vi "Initialize.vi"(8 "error in (no error)":errorcluster, 11 "NHRDCPower in":refnum<class "NHRDCPower.lvclass">) -> (0 "error out":errorcluster, 3 "NHRDCPower out":refnum<class "NHRDCPower.lvclass">)   [LabVIEW 2018, in "AcPwrPlugins.lvlib" / "NHRDCPower.lvclass"]
doc: "This VI establishes communication to the instrument and may provide other functions such as reseting the instrument or providing a range check."
uses:
  NHRDCPower.lvclass
  <instrlib>/NHRDCPowerModule/NHRDCPowerModule/NHRDCPowerModule.lvlib
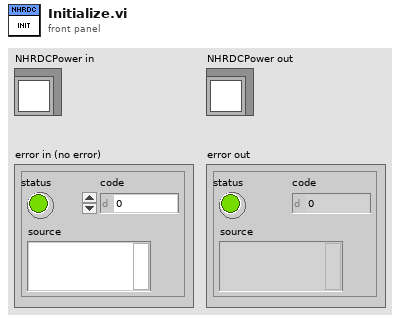
[diagram p1: front panel]
types:
  T1 = cluster{"f":bool, "instrument handle out":refnum<visa-resource-name>}[]
  T2 = typedef "AcPwrPlugins.lvlib/NHRDCPower.lvclass/Device(s)Settings.ctl" = cluster{"MeasName":string, "Modules":T3}
  T3 = typedef "AcPwrPlugins.lvlib/NHRDCPower.lvclass/Modules.ctl" = cluster{"Handle":string, "Name":string, "id query (Yes)":bool, "reset device (Yes)":bool, "Connected":bool, "Initial Battery Detect Voltage (0)":dbl, "SafetySettings":cluster{"SetWatchDog?":bool, "Voltage (V)":dbl, "Current (A)":dbl, "Power (W)":dbl, "Voltage Delay (s)":dbl, "Current Delay (s)":dbl, "Power Delay (s)":dbl}, "Options String":string, "Aperture Time (s)":dbl, "operating state (Off)":i32, "OutputSettings":cluster{"Voltage (V)":dbl, "Current (A)":dbl, "Resistance (Ohms)":dbl, "Power (W)":dbl, "Enable Voltage":bool, "Enable Current":bool, "Enable Resistance":bool, "Enable Power":bool, "Macro After Step Delay  (s)":dbl, "Wait Value (V, A, W)":dbl, "Enable Wait":bool, "Wait on Value":i32}[], "SlewRate":cluster{"Set Voltage Rate V/S":dbl, "Set Current Rate A/S":dbl, "Set Resistance Rate R/S":dbl, "Set Power Rate W/S":dbl}, "Macro":cluster{"Save Macro?":bool, "Load Macro From File?":bool, "Run Macro Continuously?":bool, "Use Macros?":bool, "Load Macro File Path":string, "Save Macro File Path":string}, "Regulation Gain (1=100%)":dbl, "UpdatingOntheFly":bool}[]
  T4 = typedef "AcPwrPlugins.lvlib/NHRDCPower.lvclass/Measurements.ctl" = cluster{"Handle":string, "Name":string, "Enabled":bool, "Measurement Value":sgl, "Measurement Type":enum16{"Power", "Current", "Voltage"}}[]
  T5 = cluster{"Handle Connected?":bool, "Instrument Handle":refnum<visa-resource-name>}
  T6 = cluster{"Handle Connected?":bool, "Instrument Handle":refnum<visa-resource-name>}[]
  T7 = cluster{"Handle":string, "Name":string, "id query (Yes)":bool, "reset device (Yes)":bool, "Connected":bool, "Initial Battery Detect Voltage (0)":dbl, "SafetySettings":cluster{"SetWatchDog?":bool, "Voltage (V)":dbl, "Current (A)":dbl, "Power (W)":dbl, "Voltage Delay (s)":dbl, "Current Delay (s)":dbl, "Power Delay (s)":dbl}, "Options String":string, "Aperture Time (s)":dbl, "operating state (Off)":i32, "OutputSettings":cluster{"Voltage (V)":dbl, "Current (A)":dbl, "Resistance (Ohms)":dbl, "Power (W)":dbl, "Enable Voltage":bool, "Enable Current":bool, "Enable Resistance":bool, "Enable Power":bool, "Macro After Step Delay  (s)":dbl, "Wait Value (V, A, W)":dbl, "Enable Wait":bool, "Wait on Value":i32}[], "SlewRate":cluster{"Set Voltage Rate V/S":dbl, "Set Current Rate A/S":dbl, "Set Resistance Rate R/S":dbl, "Set Power Rate W/S":dbl}, "Macro":cluster{"Save Macro?":bool, "Load Macro From File?":bool, "Run Macro Continuously?":bool, "Use Macros?":bool, "Load Macro File Path":string, "Save Macro File Path":string}, "Regulation Gain (1=100%)":dbl, "UpdatingOntheFly":bool}
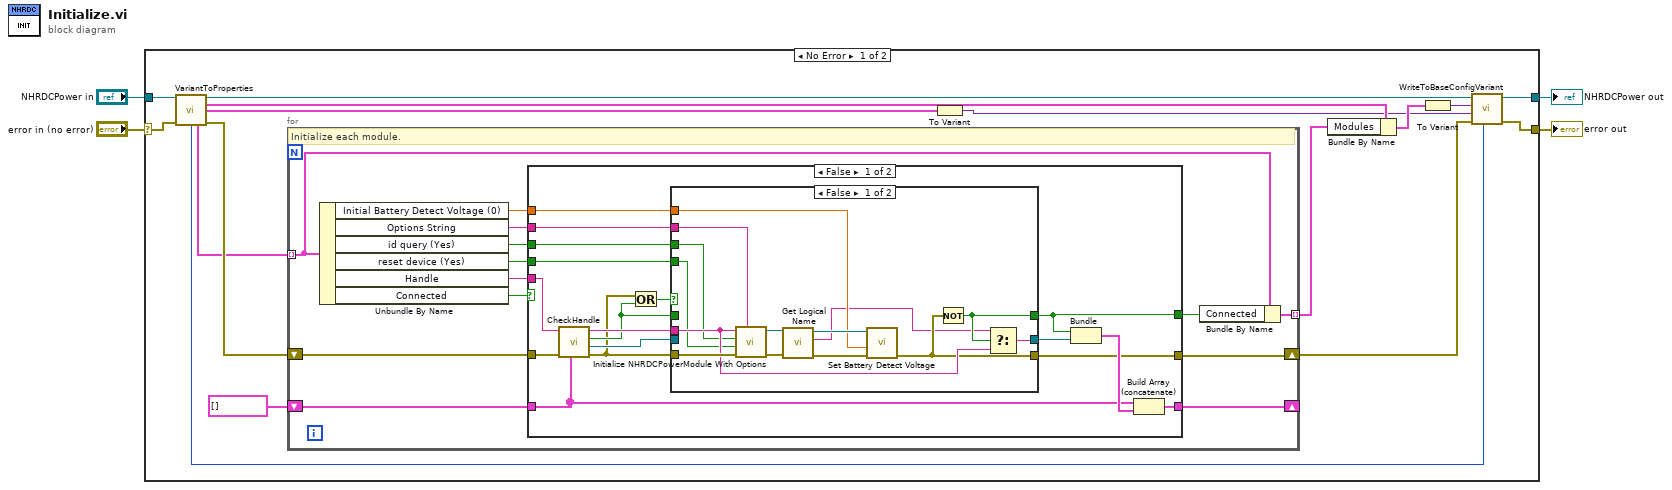
[diagram p0: block diagram]
diagram:
  n1 = case shown="No Error" "error in (no error)" {
    selector: "error in (no error)" -> [w18 w71]
    tunnel: "NHRDCPower in" -> [w17 w72]
    tunnel: [w14 w72] -> w2
    tunnel: [w13 w71] -> w1
    frame No Error {
      n2 = call "VariantToProperties.vi"("NHRDCPower in"=w17, "error in (no error)"=w18) -> ("NHRDCPower out"=w15:refnum<class "NHRDCPower.lvclass">, "NHRDC"=w11:T2, "Meas"=w5:T4, "Measurement Refresh Time (ms)"=w8:u32, "Modules"=w12:T3, "error out"=w19:errorcluster)  [unwired: 7 in, 1 out]
      n3 = for {
        shift-right: [w32] -> w16
        shift-left: w19 -> [w33]
        tunnel: w12 -> [w26] mode=indexing
        shift-right: [w30] -> _
        shift-left: T1 [] -> [w31]
        tunnel: [w25] -> w10 mode=indexing
        # "Initialize each module."
        n4 = Unbundle By Name(w26) -> ("Initial Battery Detect Voltage (0)"=w21:dbl, "Options String"=w22:string, "id query (Yes)"=w24:bool, "reset device (Yes)"=w23:bool, "Handle"=w29:string, "Connected"=w28:bool)
        n5 = case shown="False" w28 {
          selector: w28 -> [_ w70]
          tunnel: [w45 w70] -> w27
          tunnel: w29 -> [w40 _]
          tunnel: [w46 w69] -> w32
          tunnel: w33 -> [w39 w69]
          tunnel: w31 -> [w36 w68]
          tunnel: [w49 w68] -> w30
          tunnel: w24 -> [w44 _]
          tunnel: w23 -> [w43 _]
          tunnel: w22 -> [w42 _]
          tunnel: w21 -> [w34 _]
          frame False {
            n6 = call "CheckHandle.vi"("Array"=w36, "Error In"=w39, "Handle In"=w40) -> ("Error Out"=w35:errorcluster, "Instrument Handle"=w41:refnum<visa-resource-name>, "Handle Connected?"=w37:bool, "Handle Out"=w38:string)  [unwired: 5 in]
            n7 = Or(x=w35, y=w37) -> (x .or. y?=w50:bool)
            n8 = case shown="False" w50 {
              tunnel: [w63 w66] -> w45
              tunnel: w38 -> [w61 _]
              tunnel: w35 -> [w62 w67]
              tunnel: [w54 w67] -> w46
              tunnel: w37 -> [_ w66]
              tunnel: [w64 w65] -> w48
              tunnel: w41 -> [_ w65]
              tunnel: w44 -> [w60 _]
              tunnel: w43 -> [w59 _]
              tunnel: w42 -> [w57 _]
              tunnel: w34 -> [w52 _]
              frame False {
                n9 = call <instrlib>:"Initialize NHRDCPowerModule With Options.vi"("options"=w57, "error in (no error)"=w62, "reset device (Off)"=w59, "id query (Off)"=w60, "resource name"=w61) -> ("error out"=w58:errorcluster, "instrument handle out"=w56:refnum<visa-resource-name>)  [unwired: 5 in]
                n10 = call <instrlib>:"Get Logical Name.vi"("error in (no error)"=w58, "instrument handle"=w56) -> ("error out"=w55:errorcluster, "logical name"=w51:string, "instrument handle out"=w53:refnum<visa-resource-name>)  [unwired: 7 in]
                n11 = call <instrlib>:"Set Battery Detect Voltage.vi"("error in (no error)"=w55, "minimum voltage (4.0)"=w52, "instrument handle"=w53) -> ("error out"=w54:errorcluster)  [unwired: 7 in, 1 out]
                n12 = Not(x=w54) -> (.not. x?=w63:bool)
                n13 = Select(t=w51, s=w63, f=w61) -> (s? t:f=w64:string)
              }
              frame True {
              }
            }
            n14 = Bundle("Handle Connected?"=w45, "Instrument Handle"=w48) -> (w47:T5)  [unwired: 1 in]
            n15 = Build Array (concatenate)(w36, w47) -> (w49:T6)
          }
          frame True {
          }
        }
        n16 = Bundle By Name(cluster=w26, "Connected"=w27) -> (w25:T7)
      }
      n17 = To Variant(anything=w5) -> (Variant=w6:variant)
      n18 = Bundle By Name(cluster=w11, "Modules"=w10) -> (w9:T2)
      n19 = To Variant(anything=w9) -> (Variant=w7:variant)
      n20 = call "WriteToBaseConfigVariant.vi"("Measurement Refresh Time (ms)"=w8, "error in (no error)"=w16, "Meas"=w6, "Config"=w7, "NHRDCPower in"=w15) -> ("error out"=w13:errorcluster, "NHRDCPower out"=w14:refnum<class "NHRDCPower.lvclass">)  [unwired: 5 in]
    }
    frame Error {
    }
  }
  "error out" <- w1
  "NHRDCPower out" <- w2
